vi "Pre Launch Init.vi"(11 "DAQ_Module in":refnum<class "DAQ_Module.lvclass">) -> (0 "error out":errorcluster, 3 "DAQ_Module out":refnum<class "DAQ_Module.lvclass">)   [LabVIEW 2025, in "DAQ_Module.lvlib" / "DAQ_Module.lvclass"]
doc: "<p>(<strong>Filename</strong>: <span class=\"dnl\">Actor Framework.lvlib:Actor.lvclass:Pre Launch Init.vi</span>)</p>\n<p>Defines behavior that occurs after the <a href=\"nihelplauncher://docs/csh?context=lvcore_lvcomm_af_launch_nested_actor\">Launch Nested Actor</a> method is invoked but before the actor's Actor Core method begins running.</p>\n<p>By default, this method does nothing. A descendant class may override it to define behavior.</p>"
uses:
  DAQ_Module.lvclass
  DAQ_Module.lvclass/DAQ_Module.ctl
  Read ModuleName.vi
  <vilib>/ActorFramework/Actor/Actor.lvclass
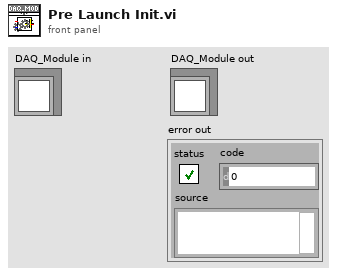
[diagram p1: front panel]
types:
  T1 = typedef "DAQ_Module.lvlib/DAQ_Module.lvclass/DAQ_Config.ctl" = map{string, T2}
  T2 = typedef "DAQ_Module.lvlib/DAQ_Module.lvclass/DAQ_Task_Config.ctl" = cluster{"TaskType":T3, "PhysicalChannels":string, "SampleRateConfiguration":cluster{"SampleRate":dbl, "SamplesPerChannel":u32, "SamplesPerRead":u32, "SampleMode":i32, "Clock Source":string}, "ChannelConfig":string}
  T3 = typedef "DAQ_Module.lvlib/DAQ_Module.lvclass/DAQ_Task_Type.ctl" = enum16{"AI", "Linear", "Angular", "AO"}
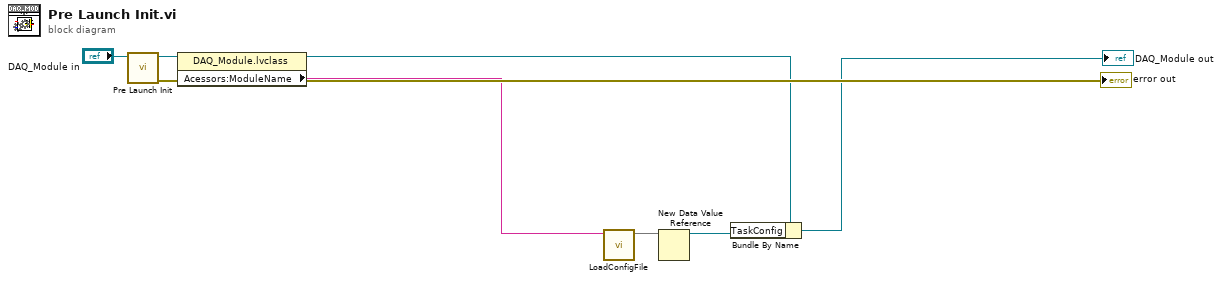
[diagram p0: block diagram]
diagram:
  n1 = call-parent "Pre Launch Init.vi"("Actor in"="DAQ_Module in") -> ("error out"=→"error out":errorcluster, "Actor out"=w6:refnum<class "DAQ_Module.lvclass">)  [unwired: 9 in]
  n2 = property class="DAQ_Module.lvclass"(reference=w6) -> (reference out=w3:refnum<class "DAQ_Module.lvclass">, "Acessors:ModuleName"=w1:string)  [unwired: 1 in, 1 out]
  n3 = call "LoadConfigFile.vi"("Model Name"=w1) -> ("Data out"=w2:T1)  [unwired: 9 in, 1 out]
  n4 = New Data Value Reference(data value=w2) -> (data value reference=w5:refnum<data-value>)  [unwired: 1 in, 1 out]
  n5 = Bundle By Name(cluster=w3, "TaskConfig"=w5) -> (→"DAQ_Module out":refnum<class "DAQ_Module.lvclass">)
